vi "Spike Remover.vi"(11 "In":dbl[](array[numeric])) -> (2 "Numeric":dbl, 3 "Out":dbl[](array[numeric]))   [LabVIEW 2017]
uses:
  <vilib>/Analysis/baseanly.llb/Mean (DBL).vi
  <vilib>/Analysis/NI_AALBase.lvlib
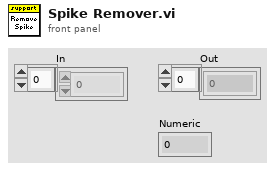
[diagram p1: front panel]
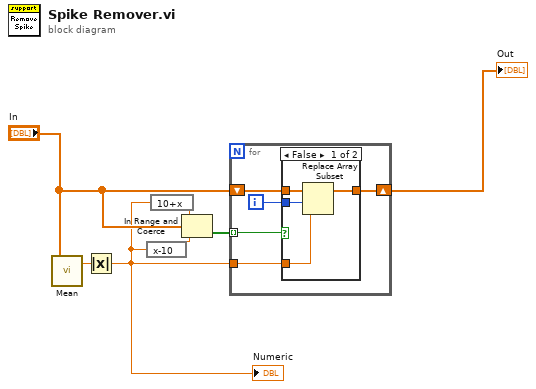
[diagram p0: block diagram]
diagram:
  n1 = call-poly <vilib>:"Mean.vi"("X"="In") -> ("mean"=w3:dbl)  [unwired: 1 out]
  n2 = Absolute Value(x=w3) -> (abs(x)=w5:dbl)
  "Numeric" <- w5
  n3 = expression code="x-10"(w5) -> (w2:dbl)
  n4 = expression code="10+x"(w5) -> (w1:dbl)
  n5 = In Range and Coerce(upper limit=w1, x="In", lower limit=w2) -> (In Range?=w4:bool[])  [unwired: 1 out]
  n6 = for {
    tunnel: w4 -> [w12] mode=indexing
    shift-right: [w10] -> w6
    shift-left: "In" -> [w11]
    tunnel: w5 -> [w8]
    i -> [w9]
    n7 = case shown="False" w12 {
      tunnel: w11 -> [w16 w17]
      tunnel: [w15 w17] -> w10
      tunnel: w9 -> [w13 _]
      tunnel: w8 -> [w14 _]
      frame False {
        n8 = Replace Array Subset(array=w16, new element=w14, index=w13) -> (w15:dbl[])
      }
      frame True {
      }
    }
  }
  "Out" <- w6
